vi "Unregister Initialize.vi"(8 "error in (no error)":errorcluster, 10 "View Enqueuer":refnum<class "Message Enqueuer.lvclass">, 11 "Create Project Model in":refnum<class "Create Project Model.lvclass">) -> (0 "error out":errorcluster, 3 "Create Project Model out":refnum<class "Create Project Model.lvclass">)   [LabVIEW 2013, in "Create Project Model.lvlib" / "Create Project Model.lvclass"]
uses:
  Create Project Model.lvclass
  <vilib>/ActorFramework/Message Enqueuer/Message Enqueuer.lvclass
  Create Project Model.lvclass/Create Project Model.ctl
  <vilib>/ActorFrameworkMVC/View Observer/View Registry/View Registry.lvclass
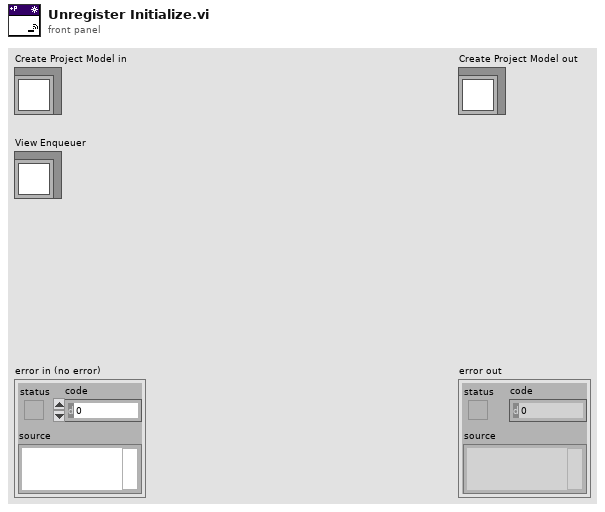
[diagram p1: front panel]
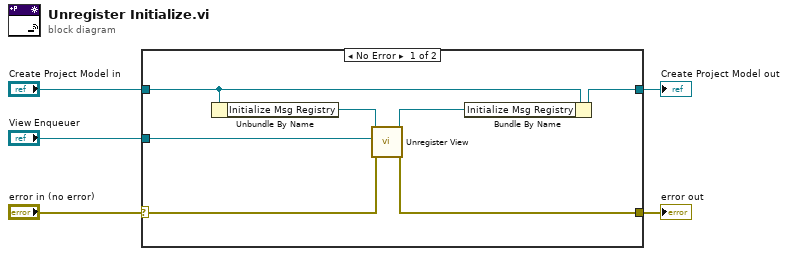
[diagram p0: block diagram]
diagram:
  n1 = case shown="No Error" "error in (no error)" {
    selector: "error in (no error)" -> [w10 w14]
    tunnel: "View Enqueuer" -> [w8 _]
    tunnel: "Create Project Model in" -> [w12 w13]
    tunnel: [w11 w13] -> w1
    tunnel: [w9 w14] -> w3
    frame No Error {
      n2 = Unbundle By Name(w12) -> ("Initialize Msg Registry"=w7:refnum<class "View Registry.lvclass">)
      n3 = call <vilib>:"Unregister View.vi"("error in (no error)"=w10, "View Enqueuer"=w8, "View Registry in"=w7) -> ("error out"=w9:errorcluster, "View Registry out"=w6:refnum<class "View Registry.lvclass">)  [unwired: 7 in]
      n4 = Bundle By Name(cluster=w12, "Initialize Msg Registry"=w6) -> (w11:refnum<class "Create Project Model.lvclass">)
    }
    frame Error {
    }
  }
  "error out" <- w3
  "Create Project Model out" <- w1
